vi "Get System Exec Text.vi"(8 "error in (no error)":errorcluster, 11 "hWnd":u32) -> (0 "error out":errorcluster, 3 "Clipboard:Read From Clipboard":string)   [LabVIEW 2013]
uses:
  USER32.DLL
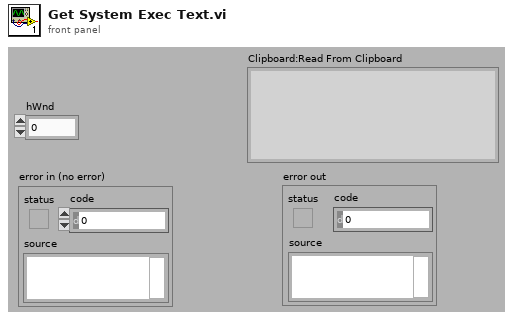
[diagram p1: front panel]
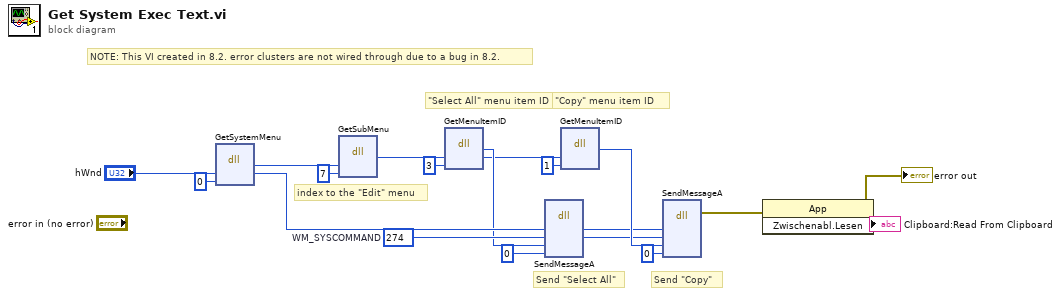
[diagram p0: block diagram]
diagram:
  w15 = u32 274  # WM_SYSCOMMAND
  # "\"Copy\" menu item ID"
  # "Send \"Copy\""
  # "\"Select All\" menu item ID"
  # "Send \"Select All\""
  # "index to the \"Edit\" menu"
  # "NOTE: This VI created in 8.2. error clusters are not wired through due to a bug in 8.2."
  n1 = dll-call lib="USER32.DLL" fn="GetSystemMenu"("hWnd"="hWnd", "bRevert"=0) -> ("hMenu"=w18:i32, "hWnd"=w16:u32)  [unwired: 4 in, 2 out]
  n2 = dll-call lib="USER32.DLL" fn="GetSubMenu"("hMenu"=w18, "nPos"=7) -> ("hMenu"=w14:i32)  [unwired: 5 in, 2 out]
  n3 = dll-call lib="USER32.DLL" fn="GetMenuItemID"("hMenu"=w14, "nPos"=3) -> ("itemID"=w12:i32, "hMenu"=w9:i32)  [unwired: 4 in, 2 out]
  n4 = dll-call lib="USER32.DLL" fn="SendMessageA" label="SendMessage"("hWnd"=w16, "msg"=w15, "wParam"=w12, "lParam"=0) -> ("hWnd"=w6:u32, "msg"=w5:u32)  [unwired: 6 in, 2 out]
  n5 = dll-call lib="USER32.DLL" fn="GetMenuItemID"("hMenu"=w9, "nPos"=1) -> ("itemID"=w7:i32)  [unwired: 5 in, 2 out]
  n6 = dll-call lib="USER32.DLL" fn="SendMessageA" label="SendMessage"("hWnd"=w6, "msg"=w5, "wParam"=w7, "lParam"=0) -> (error out=w1:errorcluster)  [unwired: 8 in, 1 out]
  n7 = invoke class="App" method="Zwischenabl.Lesen"(error in=w1) -> (error out=→"error out":errorcluster, "Read Clipbrd"=→"Clipboard:Read From Clipboard":string)  [unwired: 2 in, 1 out]
